vi "Create.vi"(8 "error in (no error)":errorcluster, 10 "Group Config":refnum<class "Group Config.lvclass">) -> (0 "error out":errorcluster, 3 "Group Buffer DBL out":refnum<class "Group Buffer DBL.lvclass">)   [LabVIEW 2020, in "VolatusHistorian.lvlib" / "Group Buffer DBL.lvclass"]
uses:
  Group Buffer DBL.lvclass
  Group Buffer DBL.lvclass/Group Buffer DBL.ctl
  VolatusConfig/Group/Group Config.lvclass
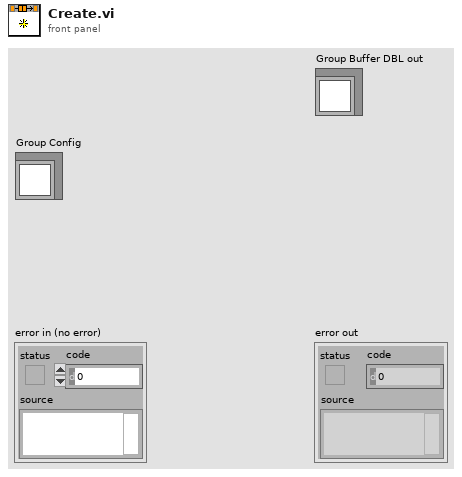
[diagram p1: front panel]
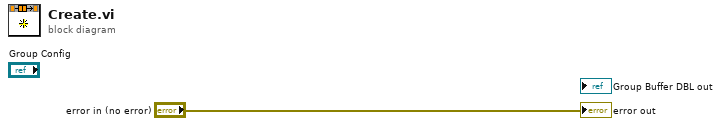
[diagram p0: block diagram]
diagram:
  "error out" <- "error in (no error)"
